vi "sequencetett.vi"() -> ()   [LabVIEW 2009]
panel:
  in  "OK Button":bool
  out "Image":T1(plugin-control)
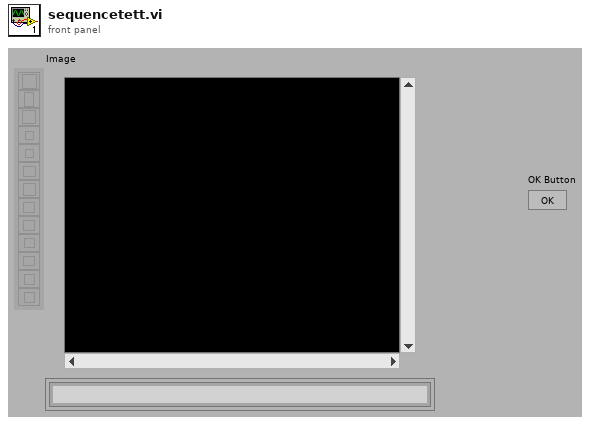
[diagram p1: front panel]
types:
  T1 = typedef "IMAQ Image.ctl" = refnum<image>
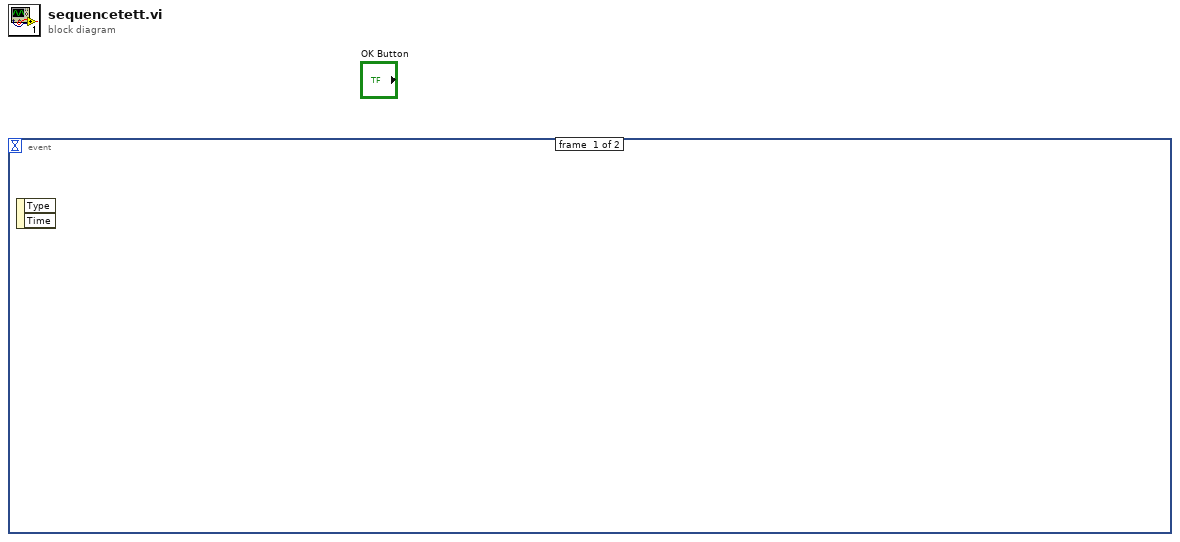
[diagram p0: block diagram]
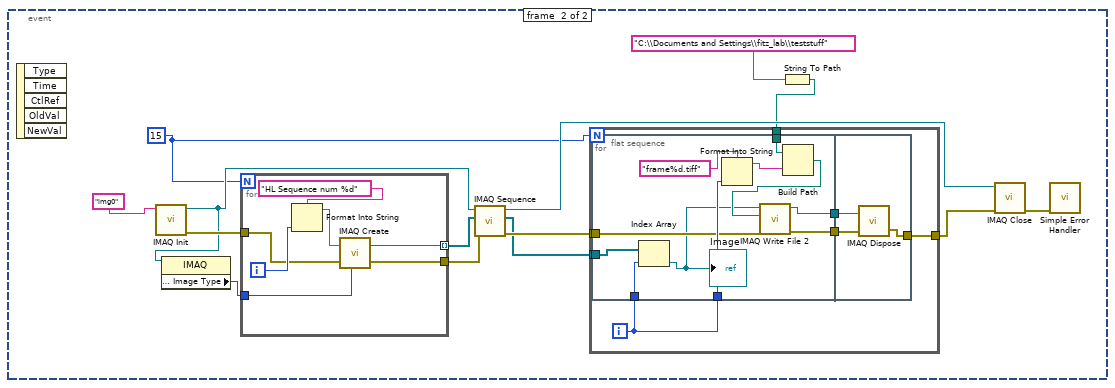
[diagram p2: hidden frame]
diagram:
  n1 = event shown="[1] \"OK Button\": Value Change" {
    selector: _ -> [_ _]
    dyn-events: _ -> [_ _]
    timeout: _ -> [_ _]
    event #0 {
      n2 = event-data() -> ()  [unwired: 1 in, 2 out]
    }
    event #1 {
      w1 = 15
      n3 = event-data() -> ()  [unwired: 1 in, 5 out]
      n4 = call <vilib>:"IMAQ Init.vi"("Interface Name"="img0") -> ("error out"=w7:errorcluster, "IMAQ Session Out"=w5:refnum<k11>)  [unwired: 9 in]
      n5 = property class="IMAQ"(reference=w5) -> ("Image Parameters : Image Type"=w3:u32)  [unwired: 1 in, 2 out]
      n6 = for {
        N: w1 -> [_]
        tunnel: w3 -> [w39]
        tunnel: [w38] -> w4 mode=indexing
        tunnel: w7 -> [w37]
        tunnel: [w36] -> w8
        i -> [w42]
        n7 = Format Into String(format string="HL Sequence num %d", w42) -> (resulting string=w40:string)  [unwired: 2 in, 1 out]
        n8 = call "IMAQ Create"("Image Name"=w40, "Image Type"=w39, "error in (no error)"=w37) -> ("New Image"=w38:T1, "error out"=w36:errorcluster)  [unwired: 2 in]
      }
      n9 = call <vilib>:"IMAQ Sequence.vi"("error in (no error)"=w8, "Images In"=w4, "IMAQ Session In"=w5) -> ("error out"=w14:errorcluster, "Images Out"=w6:T1[], "IMAQ Session Out"=w13:refnum<k11>)  [unwired: 6 in]
      n10 = String To Path(string="C:\\Documents and Settings\\fitz_lab\\teststuff") -> (path=w10:path)
      n11 = for {
        N: w1 -> [_]
        tunnel: w6 -> [w20]
        tunnel: [w18] -> w11
        tunnel: w10 -> [w21]
        tunnel: w14 -> [w16]
        i -> [w15]
        n12 = flat-sequence {
          tunnel: w21 -> [w32]
          tunnel: w15 -> [w31]
          tunnel: w20 -> [w23]
          tunnel: [w27] -> w19
          tunnel: [w26] -> w17
          tunnel: w16 -> [w25]
          tunnel: w15 -> [w24]
          tunnel: w19 -> [w35]
          tunnel: [w34] -> w18
          tunnel: w17 -> [w33]
          frame #0 {
            n13 = Index Array(array=w23, index=w24) -> (element=w22:T1)
            "Image" <- w22
            n14 = Format Into String(format string="frame%d.tiff", w31) -> (resulting string=w29:string)  [unwired: 2 in, 1 out]
            n15 = Build Path(base path=w32, name or relative path=w29) -> (appended path=w28:path)
            n16 = call-poly "IMAQ Write File 2"("error in (no error)"=w25, "File Path"=w28, "Image"=w22) -> ("error out"=w27:errorcluster, "Image Out (duplicate)"=w26:T1)  [unwired: 7 in]
          }
          frame #1 {
            n17 = call "IMAQ Dispose"("Image"=w33, "error in (no error)"=w35) -> ("error out"=w34:errorcluster)  [unwired: 4 in]
          }
        }
      }
      n18 = call <vilib>:"IMAQ Close.vi"("error in (no error)"=w11, "IMAQ Session In"=w13) -> ("error out"=w12:errorcluster)  [unwired: 9 in]
      n19 = call <vilib>:"Simple Error Handler.vi"("error in (no error)"=w12) -> ()  [unwired: 4 in, 5 out]
    }
  }
